vi "Set_Output_Voltages.vi"() -> ()   [LabVIEW 2013]
panel:
  in  "Output 2":bool
  in  "Output 1":bool
  in  "Value 2":dbl
  in  "Value 1":dbl
  in  "Range 2":dbl
  in  "Range 1":dbl
  in  "GPIB (t) / RS-232 (f)":bool
  out "error out":errorcluster
  in  "error in (no error)":errorcluster
  out "VISA resource name out":refnum<visa-resource-name>
  in  "VISA resource name":refnum<visa-resource-name>
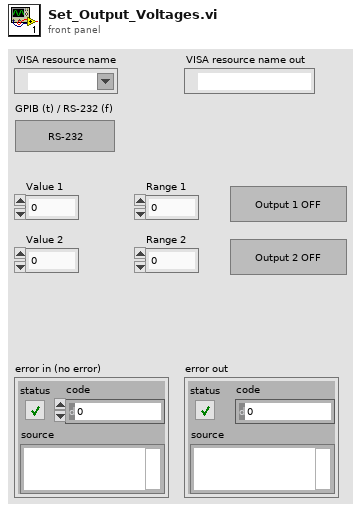
[diagram p1: front panel]
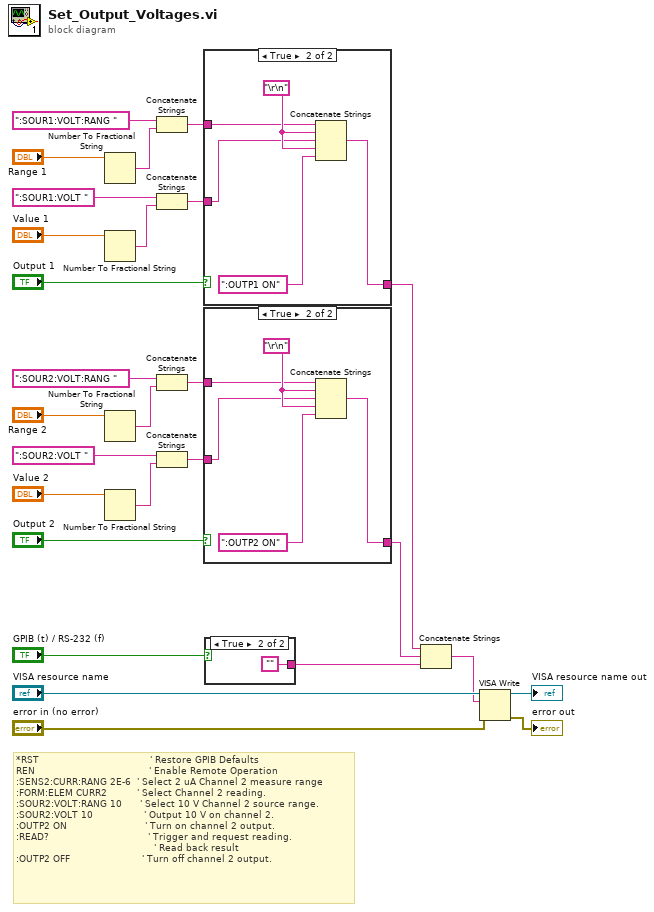
[diagram p0: block diagram]
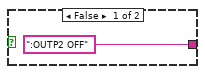
[diagram p2: hidden frame]
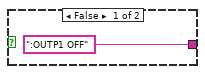
[diagram p3: hidden frame]
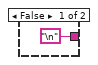
[diagram p4: hidden frame]
diagram:
  # "*RST \t\t\t                                 ' Restore GPIB Defaults\nREN                                      ' Enable Remote Operation\n:SENS2:CURR:RANG 2E-6 \t' Select 2 uA Channel 2 measure range\n:FORM:ELEM CURR2 \t        ' Select Channel 2 reading.\n:SOUR2:VOLT:RANG 10 \t    ' Select 10 V Channel 2 source range.\n:SOUR2:VOLT 10 \t\t              ' Output 10 V on channel 2.\n:OUTP2 ON \t\t                       ' Turn on channel 2 output.\n:READ? \t\t\t                             ' Trigger and request reading.\n\t\t\t                                           ' Read back result\n:OUTP2 OFF \t\t                     ' Turn off channel 2 output."
  n1 = Number To Fractional String(number="Range 1") -> (F-format string=w19:string)  [unwired: 3 in]
  n2 = Number To Fractional String(number="Value 1") -> (F-format string=w16:string)  [unwired: 3 in]
  n3 = Number To Fractional String(number="Range 2") -> (F-format string=w7:string)  [unwired: 3 in]
  n4 = Number To Fractional String(number="Value 2") -> (F-format string=w8:string)  [unwired: 3 in]
  n5 = Concatenate Strings(":SOUR1:VOLT:RANG ", w19) -> (w13:string)
  n6 = Concatenate Strings(":SOUR1:VOLT ", w16) -> (w14:string)
  n7 = Concatenate Strings(":SOUR2:VOLT:RANG ", w7) -> (w5:string)
  n8 = Concatenate Strings(":SOUR2:VOLT ", w8) -> (w6:string)
  n9 = case shown="True" "Output 1" {
    tunnel: [":OUTP1 OFF" w29] -> w2
    tunnel: w14 -> [_ w31]
    tunnel: w13 -> [_ w30]
    frame False {
    }
    frame True {
      w33 = "\r\n"
      n10 = Concatenate Strings(w30, w33, w31, w33, ":OUTP1 ON") -> (w29:string)
    }
  }
  n11 = case shown="True" "Output 2" {
    tunnel: [":OUTP2 OFF" w35] -> w1
    tunnel: w6 -> [_ w37]
    tunnel: w5 -> [_ w36]
    frame False {
    }
    frame True {
      w39 = "\r\n"
      n12 = Concatenate Strings(w36, w39, w37, w39, ":OUTP2 ON") -> (w35:string)
    }
  }
  n13 = case shown="True" "GPIB (t) / RS-232 (f)" {
    tunnel: ["\n" ""] -> w3
    frame False {
    }
    frame True {
    }
  }
  n14 = Concatenate Strings(w2, w1, w3) -> (w23:string)
  n15 = VISA Write(VISA resource name="VISA resource name", write buffer=w23, error in (no error)="error in (no error)") -> (VISA resource name out=→"VISA resource name out":refnum<visa-resource-name>, error out=→"error out":errorcluster)  [unwired: 1 out]
